vi "GetAzCamToolParameter.vi"(0 "Parameter":string) -> (1 "Error":bool, 2 "Value":string)   [LabVIEW 2014]
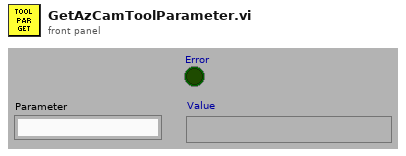
[diagram p1: front panel]
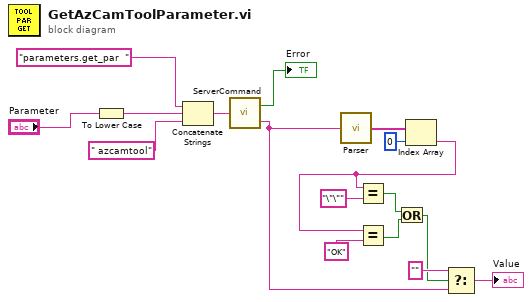
[diagram p0: block diagram]
diagram:
  n1 = To Lower Case(string="Parameter") -> (all lower case string=w2:string)
  n2 = Concatenate Strings("parameters.get_par  " ("Attribute"), w2, " azcamtool" ("string")) -> (w3:string)
  n3 = call "ServerCommand.vi"("Command"=w3) -> ("Error"=→"Error":bool, "Reply"=w11:string)
  n4 = call "Parser.vi"("string"=w11) -> ("Out Strings"=w15:string[])
  n5 = Index Array(array=w15, index=0) -> (element=w10:string)
  n6 = Equal?(x=w10, y="\"\"") -> (x = y?=w8:bool)
  n7 = Equal?(x=w10, y="OK") -> (x = y?=w7:bool)
  n8 = Or(x=w8, y=w7) -> (x .or. y?=w6:bool)
  n9 = Select(t="", s=w6, f=w11) -> (s? t:f=→"Value":string)
